vi "lvpeak_open_camera.vi"(8 "error in (no error)":errorcluster, 11 "identifier":string) -> (0 "error out":errorcluster, 3 "camera_id":u64)   [LabVIEW 2024, in "Vision.lvlib"]
uses:
  Vision.lvlib
  bin/LVPeak.dll
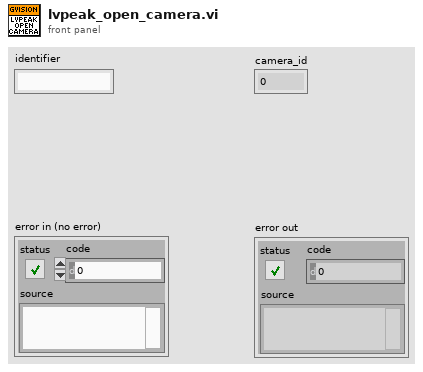
[diagram p1: front panel]
types:
  T1 = typedef "Vision.lvlib/lvpeak_camera.ctl" = cluster{"identifier":string, "camera_id":u64}
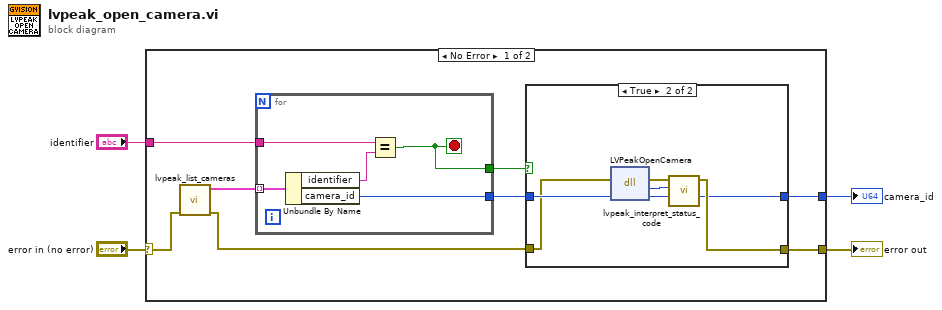
[diagram p0: block diagram]
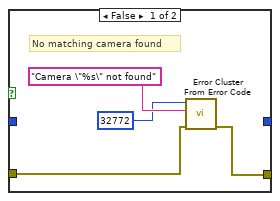
[diagram p2: hidden frame]
diagram:
  n1 = case shown="No Error" "error in (no error)" {
    selector: "error in (no error)" -> [w12 w28]
    tunnel: [w6 w28] -> w3
    tunnel: "identifier" -> [w10 _]
    tunnel: [w5 _] -> w1
    frame No Error {
      n2 = call "lvpeak_list_cameras.vi"("error in (no error)"=w12) -> ("error out"=w7:errorcluster, "LVPeak Cameras"=w11:T1[])  [unwired: 9 in]
      n3 = for {
        tunnel: w11 -> [w27] mode=indexing
        tunnel: w10 -> [w26]
        tunnel: [w24] -> w8
        tunnel: [w23] -> w9
        stop <- w23 stop-if-true
        n4 = Unbundle By Name(w27) -> ("identifier"=w25:string, "camera_id"=w24:u64)
        n5 = Equal?(x=w26, y=w25) -> (x = y?=w23:bool)
      }
      n6 = case shown="True" w9 {
        tunnel: w8 -> [_ w22]
        tunnel: w7 -> [w16 w19]
        tunnel: [w13 w18] -> w6
        tunnel: [_ w17] -> w5
        frame False {
          # "No matching camera found"
          n7 = call <vilib>:"Error Cluster From Error Code.vi"("error in (no error)"=w16, "error message (\"\")"="Camera \"%s\" not found" ("error message (\"\")"), "error code (0)"=32772) -> ("error out"=w13:errorcluster)  [unwired: 6 in]
        }
        frame True {
          n8 = dll-call lib="C:/Users/cfang/Desktop/nebraska-silicon-lab/pixel-gantry-control/Gantry/Shared Components/bin/LVPeak.dll" fn="LVPeakOpenCamera"(error in=w19, "camera_id"=w22) -> (error out=w21:errorcluster, "return type"=w20:i32, "camera_id"=w17:u64)  [unwired: 2 in, 1 out]
          n9 = call "lvpeak_interpret_status_code.vi"("status_code"=w20, "error in (no error)"=w21) -> ("error out"=w18:errorcluster)  [unwired: 9 in]
        }
      }
    }
    frame Error {
    }
  }
  "error out" <- w3
  "camera_id" <- w1
